vi "Set Disable Heater Button Ref.vi"(8 "error in (no error)":errorcluster, 10 "Disable Heater Button Ref":refnum<vi>, 11 "Thermal Chamber Controller In":refnum<class "Thermal Chamber Controller.lvclass">) -> (0 "error out":errorcluster, 3 "Thermal Chamber Controller Out":refnum<class "Thermal Chamber Controller.lvclass">)   [LabVIEW 2020, in "Thermal Chamber Controller.lvclass"]
uses:
  Thermal Chamber Controller.lvclass
  C:/Program Files (x86)/National Instruments/LabVIEW 2020/vi.lib/Asteme/Triarc Framework/Process/Process.lvclass
  <vilib>/Asteme/Triarc Framework/Process/Process.lvclass/Process.ctl
  Thermal Chamber Controller.lvclass/Thermal Chamber Controller.ctl
  <vilib>/Utility/error.llb/Clear Errors.vi
  <vilib>/Asteme/Triarc Framework/Process/Process.lvclass
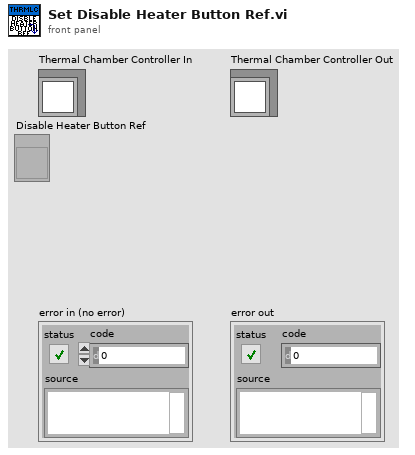
[diagram p1: front panel]
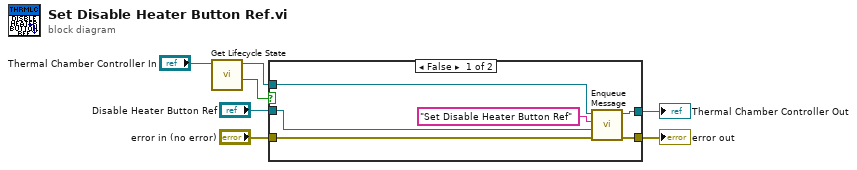
[diagram p0: block diagram]
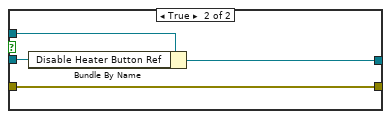
[diagram p2: hidden frame]
diagram:
  n1 = call <vilib>:"Get Lifecycle State.vi"("Process In"="Thermal Chamber Controller In") -> ("In Process Loop?"=w3:bool, "Process Out"=w6:refnum<class "Thermal Chamber Controller.lvclass">)  [unwired: 7 in, 2 out]
  n2 = case shown="False" w3 {
    tunnel: w6 -> [w13 w17]
    tunnel: [w12 w15] -> w5
    tunnel: "error in (no error)" -> [w9 w16]
    tunnel: [w10 w16] -> w4
    tunnel: "Disable Heater Button Ref" -> [w8 w14]
    frame False {
      n3 = call <vilib>:"Enqueue Message.vi"("error in (no error)"=w9, "Message Data"=w8, "Message"="Set Disable Heater Button Ref" ("API Message"), "Process In"=w13) -> ("error out"=w10:errorcluster, "Process Out"=w12:refnum<class "Thermal Chamber Controller.lvclass">)  [unwired: 6 in]
    }
    frame True {
      n4 = Bundle By Name(cluster=w17, "Disable Heater Button Ref"=w14) -> (w15:refnum<class "Thermal Chamber Controller.lvclass">)
    }
  }
  "error out" <- w4
  "Thermal Chamber Controller Out" <- w5
